vi "VFH-interpolate_align.vi"(7 "Xi":dbl[](array[numeric]), 10 "data":dbl[](array[numeric]), 11 "Frequency":dbl[](array[numeric])) -> (2 "data out":dbl[](array[numeric]), 3 "Frequency out":dbl[](array[numeric]))   [LabVIEW 2020, in "VFH-VNA_File_Handler.lvlib"]
uses:
  VFH-VNA_File_Handler.lvlib
  <vilib>/gmath/NI_Gmath.lvlib
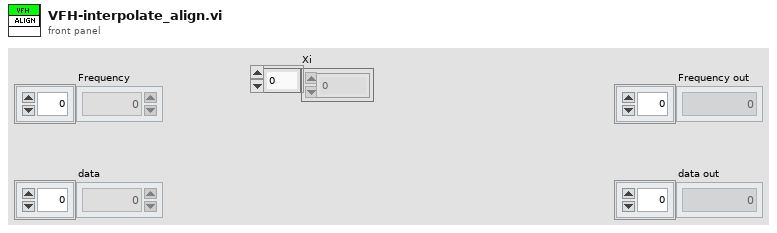
[diagram p1: front panel]
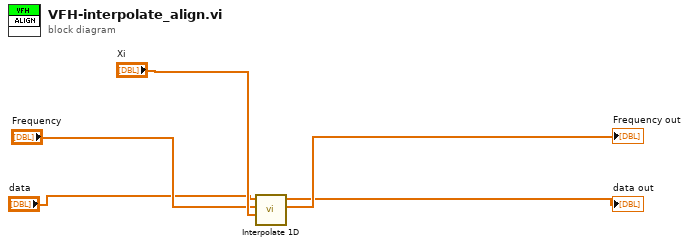
[diagram p0: block diagram]
diagram:
  n1 = call <vilib>:"Interpolate 1D.vi"("xi"="Xi", "X"="Frequency", "Y"="data") -> ("xi used"=→"Frequency out":dbl[], "yi"=→"data out":dbl[])  [unwired: 6 in, 1 out]
